vi "Part 1.vi"(11 "Input":string) -> (3 "Output":i64)   [LabVIEW 2021]
uses:
  <userlib>/_OpenG.lib/string/string.llb/Convert EOLs (String)__ogtk.vi
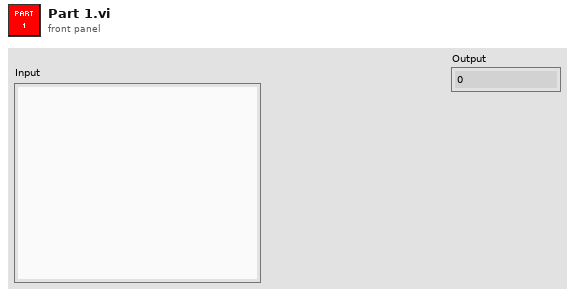
[diagram p1: front panel]
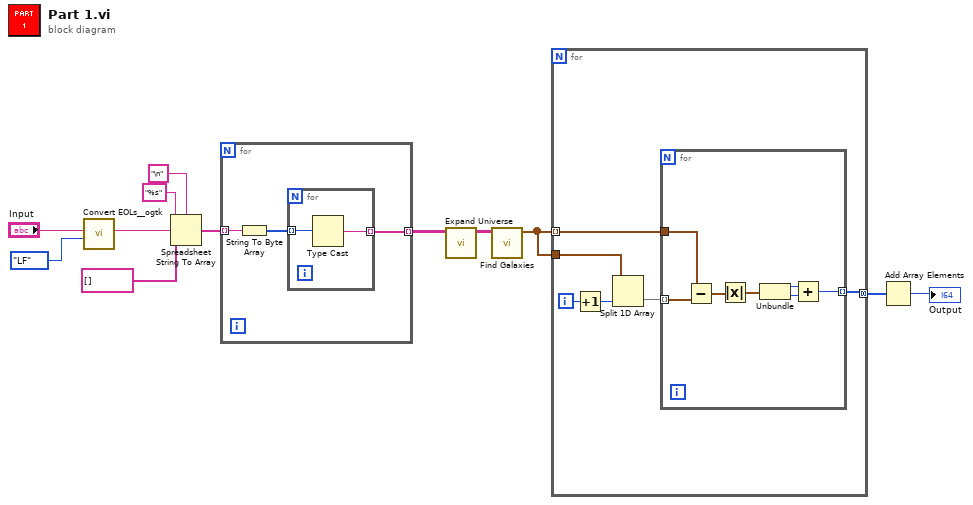
[diagram p0: block diagram]
diagram:
  n1 = call-poly <userlib>:"Convert EOLs__ogtk.vi"("Convert to:"=enum16{"CR", "LF", "CRLF"}."LF", "String in"="Input") -> ("String out"=w8:string)  [unwired: 9 in]
  n2 = Spreadsheet String To Array(delimiter (Tab)="\n", format string="%s", spreadsheet string=w8, array type (2D Dbl)=string[] []) -> (array=w6:string[])
  n3 = for {
    tunnel: w6 -> [w15] mode=indexing
    tunnel: [w13] -> w5 mode=indexing
    n4 = String To Byte Array(string=w15) -> (unsigned byte array=w14:u8[])
    n5 = for {
      tunnel: w14 -> [w17] mode=indexing
      tunnel: [w16] -> w13 mode=indexing
      n6 = Type Cast(x=w17) -> (*(type *) &x=w16:string)  [unwired: 1 in]
    }
  }
  n7 = call "Expand Universe.vi"("Univers In"=w5) -> ("Universe Out"=w4:string[][])  [unwired: 10 in]
  n8 = call "Find Galaxies.vi"("Universe In"=w4) -> ("Galaxies"=w3:cluster{"x":i32, "y":i32}[])  [unwired: 10 in]
  n9 = for {
    tunnel: w3 -> [w19] mode=indexing
    tunnel: w3 -> [w23]
    tunnel: [w18] -> w2 mode=concatenating
    i -> [w22]
    n10 = Increment(x=w22) -> (x+1=w21:i32)
    n11 = Split 1D Array(array=w23, index=w21) -> (second subarray=w20:cluster{"x":i32, "y":i32}[])  [unwired: 1 out]
    n12 = for {
      tunnel: w20 -> [w30] mode=indexing
      tunnel: w19 -> [w29]
      tunnel: [w24] -> w18 mode=indexing
      n13 = Subtract(x=w29, y=w30) -> (x-y=w28:cluster{"x":i32, "y":i32})
      n14 = Absolute Value(x=w28) -> (abs(x)=w27:cluster{"x":i32, "y":i32})
      n15 = Unbundle(w27) -> ("x"=w26:i32, "y"=w25:i32)
      n16 = Add(x=w26, y=w25) -> (x+y=w24:i32)
    }
  }
  n17 = Add Array Elements(numeric array=w2) -> (sum=→"Output":i32)
